vi "Read Histogram Data.vi"(1 "Start-Stop#":i8=1 min=1 max=4 step=1) -> (0 "Array":i64[](array[numeric]))   [LabVIEW 2012]
doc: "The Basic Serial Read and Write example performs a Serial Port Read, a Serial Port Write, or a combination of these actions. The user selects the actions (read or write) on the front panel. If both are selected, the VI will write the data first, read data, and then close the VISA session that is opened to the port. This VI will wait until the specified number of bytes is received at the port or until a termination character is read.\n\nINSTRUCTIONS:\n1) Select the serial resource and configuration parameters (baud rate, data bits, parity, stop bits, flow control).\n2) Select the operations to be performed. \n3) Connect the serial port to your device. If no device is available, perform a loopback test by doing one of the following. Short pins 2 and 3 on a RS-232 cable or short pin 4 to pin 8 and pin 5 to pin 9 on a RS-485/422 cable. \n4) Run the VI to see the data read. (The \"read string\" will match the \"string to write\" if a loopback test was performed.)\n\nNote: The parameters set for the serial port must match the parameters of the connected instrument or device. In this example, the bytes to read parameter specifies the number of bytes that the serial port reads. If there were more bytes at the port than the number specified in bytes to read, those bytes would not be read. Also, if you specify to read more bytes than the number of bytes actually read, you might receive a timeout error message.\n\nOn the block diagram, the Configure Serial Port VI sets the configuration parameters. The front panel displays the controls used to configure the basic parameters, such as baud rate, data bits, and parity. Constants configure the other parameters the user probably does not need set. After the VISA Configure Serial Port VI opens the VISA session and configures the port, the VI passes the VISA resource name to other VIs that perform operations on that VISA resource. The VISA Write function sends a command to the serial device and the VISA Read function returns data based on the command. The VISA Close function then closes the reference to the serial device. It is important to close the reference; otherwise communication through with that port through protocols other than VISA might not be possible."
uses:
  Correlator port.vi
panel:
  out "Serial Settings:Number of Bytes at Serial Port":u32
  out "read buffer":string
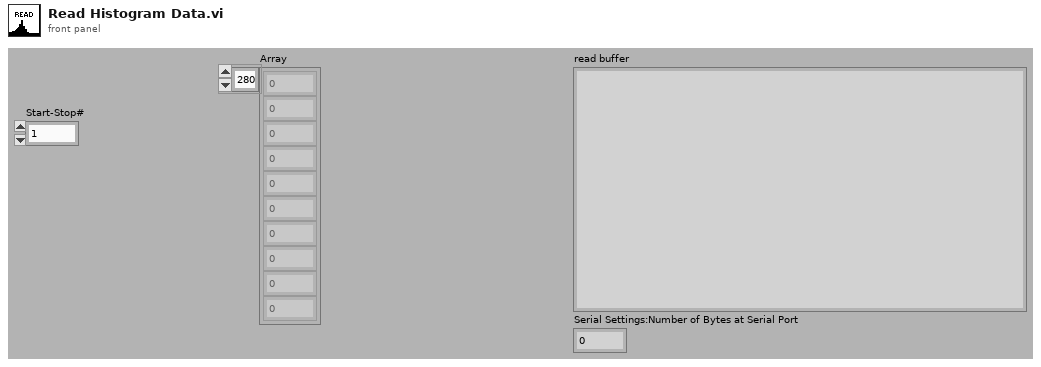
[diagram p1: front panel]
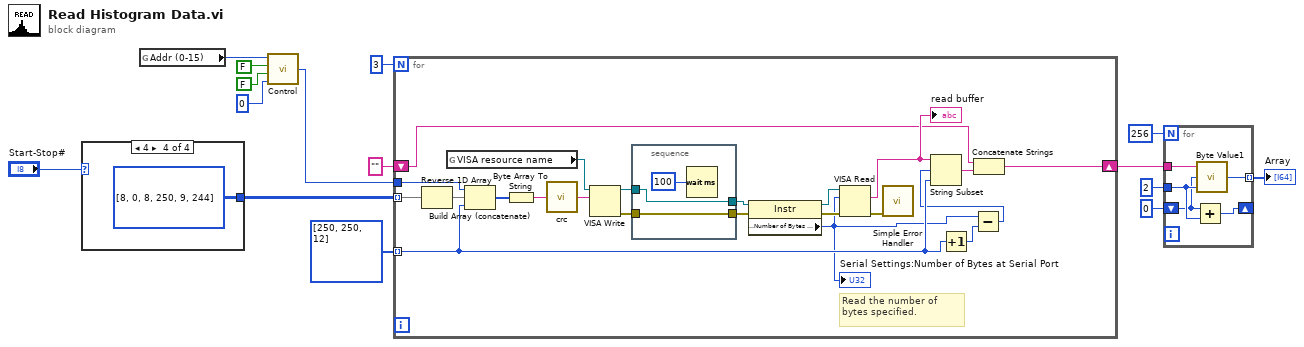
[diagram p0: block diagram]
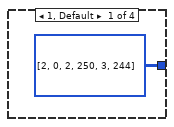
[diagram p2: hidden frame]
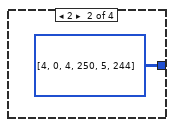
[diagram p3: hidden frame]
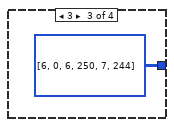
[diagram p4: hidden frame]
diagram:
  n1 = case shown="4" "Start-Stop#" {
    tunnel: [i16[][] [[2, 0], [2, 250], [3, 244]] i16[][] [[4, 0], [4, 250], [5, 244]] i16[][] [[6, 0], [6, 250], [7, 244]] i16[][] [[8, 0], [8, 250], [9, 244]]] -> w9
    frame 1, Default {
    }
    frame 2 {
    }
    frame 3 {
    }
    frame 4 {
    }
  }
  n2 = global read "Correlator port.vi" "Addr (0-15)"() -> (w8:i8)
  n3 = call "Control.vi"("Page"=i8 0, "Error"=FALSE, "Write"=FALSE, "Addr"=w8) -> ("Control Byte"=w10:u32)
  n4 = for {
    N: 3 -> [_]
    tunnel: w10 -> [w34]
    tunnel: w9 -> [w33] mode=indexing
    tunnel: i16[] [250, 250, 12] ("Offset") -> [w23] mode=indexing
    shift-right: [w25] -> w14
    shift-left: "" -> [w24]
    # "Read the number of bytes specified."
    n5 = Reverse 1D Array(array=w33) -> (reversed array=w32:i16[])
    n6 = global read "Correlator port.vi" "VISA resource name"() -> (w36:refnum<visa-resource-name>)
    n7 = Build Array (concatenate)(w34, w32, w23) -> (w31:u32[])
    n8 = Byte Array To String(unsigned byte array=w31) -> (string=w30:string)
    n9 = call "crc.vi"("Input string"=w30) -> ("Output (with crc)"=w29:string)
    n10 = VISA Write(VISA resource name=w36, write buffer=w29) -> (VISA resource name out=w39:refnum<visa-resource-name>, error out=w41:errorcluster)  [unwired: 1 in, 1 out]
    n11 = stacked-sequence {
      tunnel: w41 -> [w44]
      tunnel: [w44] -> w40
      tunnel: w39 -> [w43]
      tunnel: [w43] -> w38
      frame #0 {
        n12 = Wait (ms)(milliseconds to wait=u32 100 ("delay before read (ms)")) -> ()  [unwired: 1 out]
      }
    }
    n13 = property class="Instr"(reference=w38, error in=w40) -> (reference out=w28:refnum<visa-resource-name>, error out=w27:errorcluster, "Serial Settings:Number of Bytes at Serial Port"=w21:u32)
    "Serial Settings:Number of Bytes at Serial Port" <- w21
    n14 = VISA Read(VISA resource name=w28, byte count=w21, error in (no error)=w27) -> (read buffer=w37:string, error out=w35:errorcluster)  [unwired: 2 out]
    "read buffer" <- w37
    n15 = call <vilib>:"Simple Error Handler.vi"("error in (no error)"=w35) -> ()  [unwired: 1 in, 8 out]
    n16 = Increment(x=w23) -> (x+1=w22:i16)
    n17 = Subtract(x=w21, y=w22) -> (x-y=w20:u32)
    n18 = String Subset(string=w37, offset (0)=w20, length (rest)=w23) -> (substring=w26:string)
    n19 = Concatenate Strings(w24, w26) -> (w25:string)
  }
  n20 = for {
    N: 256 -> [_]
    tunnel: 2 ("Max Exposition Time (ms)") -> [w48]
    tunnel: w14 -> [w49]
    shift-right: [w47] -> _
    shift-left: i8 0 -> [w46]
    tunnel: [w45] -> w3 mode=indexing
    n21 = Add(x=w46, y=w48) -> (x+y=w47:i32)
    n22 = call "Byte Value1.vi"("Length"=w48, "Offset"=w46, "string"=w49) -> ("Value"=w45:i64)
  }
  "Array" <- w3
